vi "FreqPwrMeasureExample.vi"(7 "Freq":dbl=2412000000.0, 8 "ReferenceLevel":dbl, 9 "PhyPort":u16=6, 10 "Pwr/Freq":u16=1, 11 "VISA Resource Name":string="TCPIP0::10.144.41.39::inst0::INSTR") -> (3 "result":dbl=-87376.21875 format="%.6g")   [LabVIEW 2015]
uses:
  VISAOperation.ctl
  PhyPort.ctl
panel:
  out "offset past number":i32=15
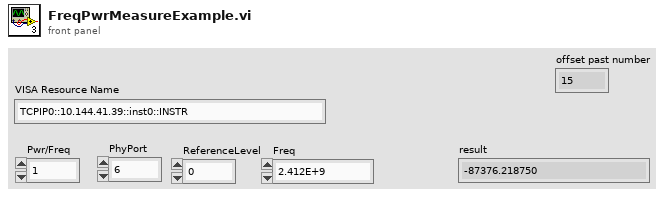
[diagram p1: front panel]
types:
  T1 = typedef "PhyPort.ctl" = enum16{"Port0", "Port1", "Port2", "Port3", "Port4", "Port5", "Port6", "Port7"}
  T2 = cluster{"TriggerSource":enum16{"RIO0", "RIO1"}, "ReferenceLevel":dbl, "Freq":dbl, "PhyPort":T1}
  T3 = typedef "VISAOperation.ctl" = enum16{"RunFile", "OpenDebugPanel", "ReadError", "ReadSTB", "Reset", "Clean", "CloseVISA", "RunCMD", "OpenVISA"}
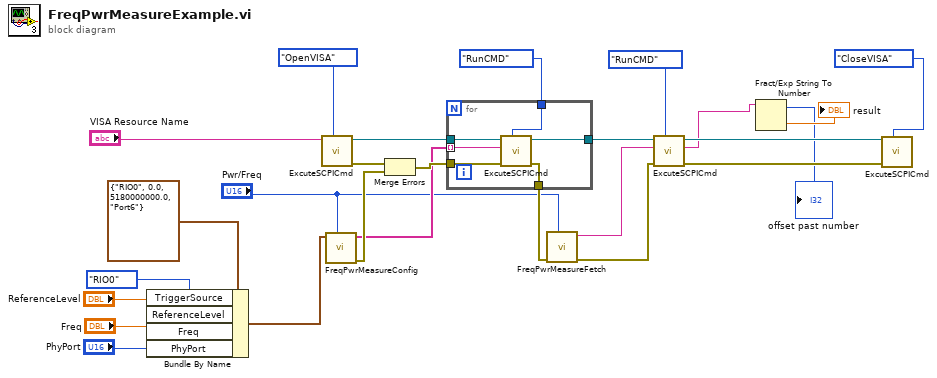
[diagram p0: block diagram]
diagram:
  n1 = Bundle By Name(cluster=T2 {"TriggerSource"=enum."RIO0", "ReferenceLevel"=0.0, "Freq"=5180000000.0, "PhyPort"=enum."Port6"} ("MeasureConfig"), "TriggerSource"=enum16{"RIO0", "RIO1"}."RIO0", "ReferenceLevel"="ReferenceLevel", "Freq"="Freq", "PhyPort"="PhyPort") -> (w8:T2)
  n2 = call "ExcuteSCPICmd.vi"("VISAOperation"=VISAOperation."OpenVISA", "VISA resource name"="VISA Resource Name") -> ("error out"=w23:errorcluster, "reference out"=w22:refnum<visa-resource-name>)  [unwired: 6 in, 2 out]
  n3 = call "FreqPwrMeasureConfig.vi"("Freq/Pwr"="Pwr/Freq", "FreqMeasureConfig"=w8) -> ("error out"=w15:errorcluster, "FreqMeasureConfig"=w12:string[])  [unwired: 8 in]
  n4 = Merge Errors(w23, w15) -> (w19:errorcluster)
  n5 = for {
    tunnel: VISAOperation."RunCMD" ("VISAOperation") -> [w30]
    tunnel: w22 -> [w32]
    tunnel: [w31] -> w21
    tunnel: w12 -> [w29] mode=indexing
    tunnel: w19 -> [w28]
    tunnel: [w27] -> w14
    n6 = call "ExcuteSCPICmd.vi"("VISAOperation"=w30, "error in (no error)"=w28, "Run Command"=w29, "VISA resource name"=w32) -> ("error out"=w27:errorcluster, "reference out"=w31:refnum<visa-resource-name>)  [unwired: 4 in, 2 out]
  }
  n7 = call "FreqPwrMeasureFetch.vi"("Freq/Pwr"="Pwr/Freq", "error in (no error)"=w14) -> ("error out"=w13:errorcluster, "FreqFetchCMD"=w16:string)  [unwired: 8 in]
  n8 = call "ExcuteSCPICmd.vi"("VISAOperation"=VISAOperation."RunCMD", "error in (no error)"=w13, "Run Command"=w16, "VISA resource name"=w21) -> ("error out"=w17:errorcluster, "Results"=w7:string, "reference out"=w18:refnum<visa-resource-name>)  [unwired: 4 in, 1 out]
  n9 = Fract/Exp String To Number(string=w7) -> (offset past number=→"offset past number":i32, number=→"result":dbl)  [unwired: 3 in]
  n10 = call "ExcuteSCPICmd.vi"("VISAOperation"=VISAOperation."CloseVISA", "error in (no error)"=w17, "VISA resource name"=w18) -> ()  [unwired: 5 in, 4 out]
